vi "AK TCP Factory Wrapper.vi"(8 "Error In":errorcluster, 10 "AK TCP Settings":T1) -> (0 "Error Out":errorcluster, 3 "AK TCP Out":refnum<class "AK TCP.lvclass">)   [LabVIEW 2018, in "Instrument Addon Scripting API.lvlib"]
uses:
  Instrument Addon Scripting API.lvlib
  Addon/Support Libraries/Protocols.lvlibp/AK TCP/AK TCP Settings.ctl
  Addon/Support Libraries/Protocols.lvlibp/AK TCP/AK TCP.lvclass
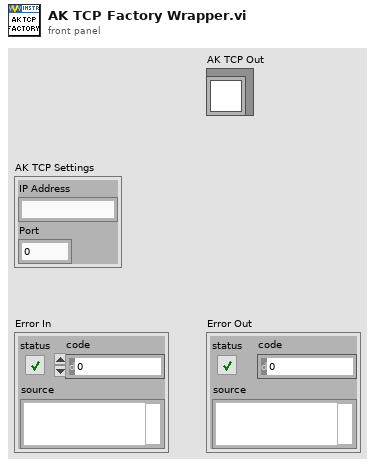
[diagram p1: front panel]
types:
  T1 = typedef "Protocols.lvlibp/AK TCP.lvclass/AK TCP Settings.ctl" = cluster{"IP Address":string, "Port":u16}
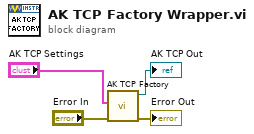
[diagram p0: block diagram]
diagram:
  n1 = call "AK TCP Factory.vi"("Error In"="Error In", "AK TCP Settings"="AK TCP Settings") -> ("Error Out"=→"Error Out":errorcluster, "AK TCP Out"=→"AK TCP Out":refnum<class "AK TCP.lvclass">)  [unwired: 8 in]
